vi "tester 2.vi"() -> ()   [LabVIEW 2020]
uses:
  VNA-Addresses.ctl
  <vilib>/Instr/_visa.llb/VISA Configure Serial Port (Instr).vi
panel:
  out "unsigned byte array 3":u8[](array[numeric])
  out "*(type *) &x 4":u64
  out "unsigned byte array 4":u8[](array[numeric]) format="%x"
  in  "byte order (0:big-endian, network order)":T1(ring)=enum."little-endian"
  out "*(type *) &x 3":u64
  out "*(type *) &x 2":u64
  in  "s":bool
  in  "unsigned byte array 2":u8[](array[numeric]) format="%x"
  out "unsigned byte array":u8[](array[numeric]) format="%x"
  out "Respons hex 2":u64 format="%x"
  out "length":i32
  out "XY Graph":cluster{i32[], dbl[]}[](graph)
  in  "y":bool
  out "Array":T2(array[cluster])
  in  "Command 2":i32 format="%x"
  in  "Write free":bool
  out "CMDADDR":u64 format="%x"
  out "*(type *) &x":u64
  out "data to write":u64 format="%x"
  in  "Read/write":bool
  in  "Address":T3
  in  "DAta to Write":u64
  out "bytes at port last":u32
  out "error out":errorcluster
  out "read buffer":string
  out "command worked":bool
  in  "clear command flag":bool
  out "Response string":string
  out "Respons hex":u64 format="%x"
  in  "Stop":bool
  in  "Write cmd":bool
  out "bytes at port":u32
  out "reading":bool
  out "Command":string="*IDN?"
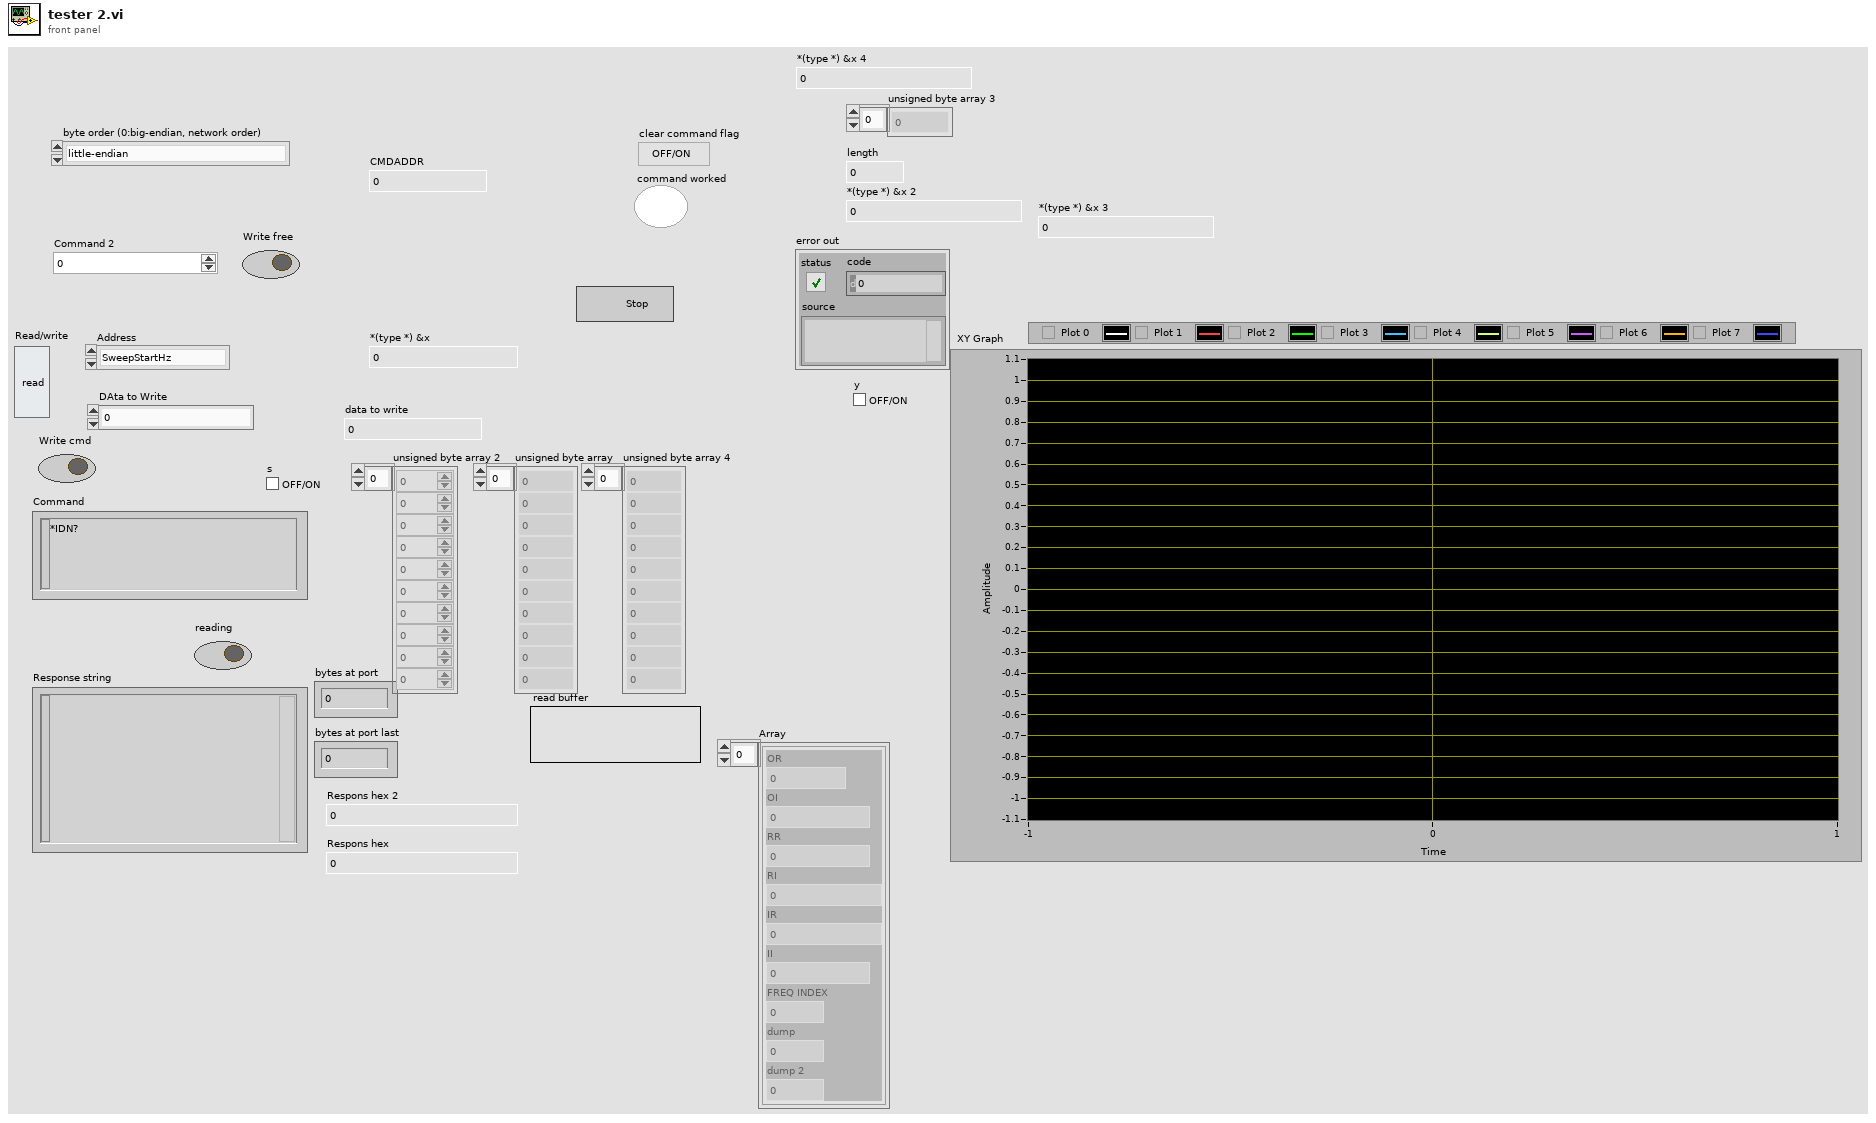
[diagram p1: front panel]
types:
  T1 = enum16{"big-endian, network order", "native, host order", "little-endian"}
  T2 = cluster{"OR":i32, "OI":i32, "RR":i32, "RI":i32, "IR":i32, "II":i32, "FREQ INDEX":u16, "dump":u16, "dump 2":u32}[]
  T3 = typedef "VNA-Addresses.ctl" = enum16{"SweepStartHz", "SweepStopHz", "SweepPoints", "valuesPerFrequency", "RawSamplesMode", "ValuesFIFO", "deviceVariant", "protocolVersion", "hardwareRevision", "firmwareMajor", "firmwareMinor"}
  T4 = cluster{"baud rate":u32, "data bits":u16, "parity":enum16{"None", "Odd", "Even", "Mark", "Space"}, "stop bits":u16, "flow control":u16}
  T5 = typedef "VNA-Commands.ctl" = enum16{"Nop", "Indicate", "Read 1B", "Read 2B", "Read 4B", "Read 8B", "Read FIFO", "Write 1B", "Write 2B", "Write 4B", "Write 8B", "Write FIFO"}
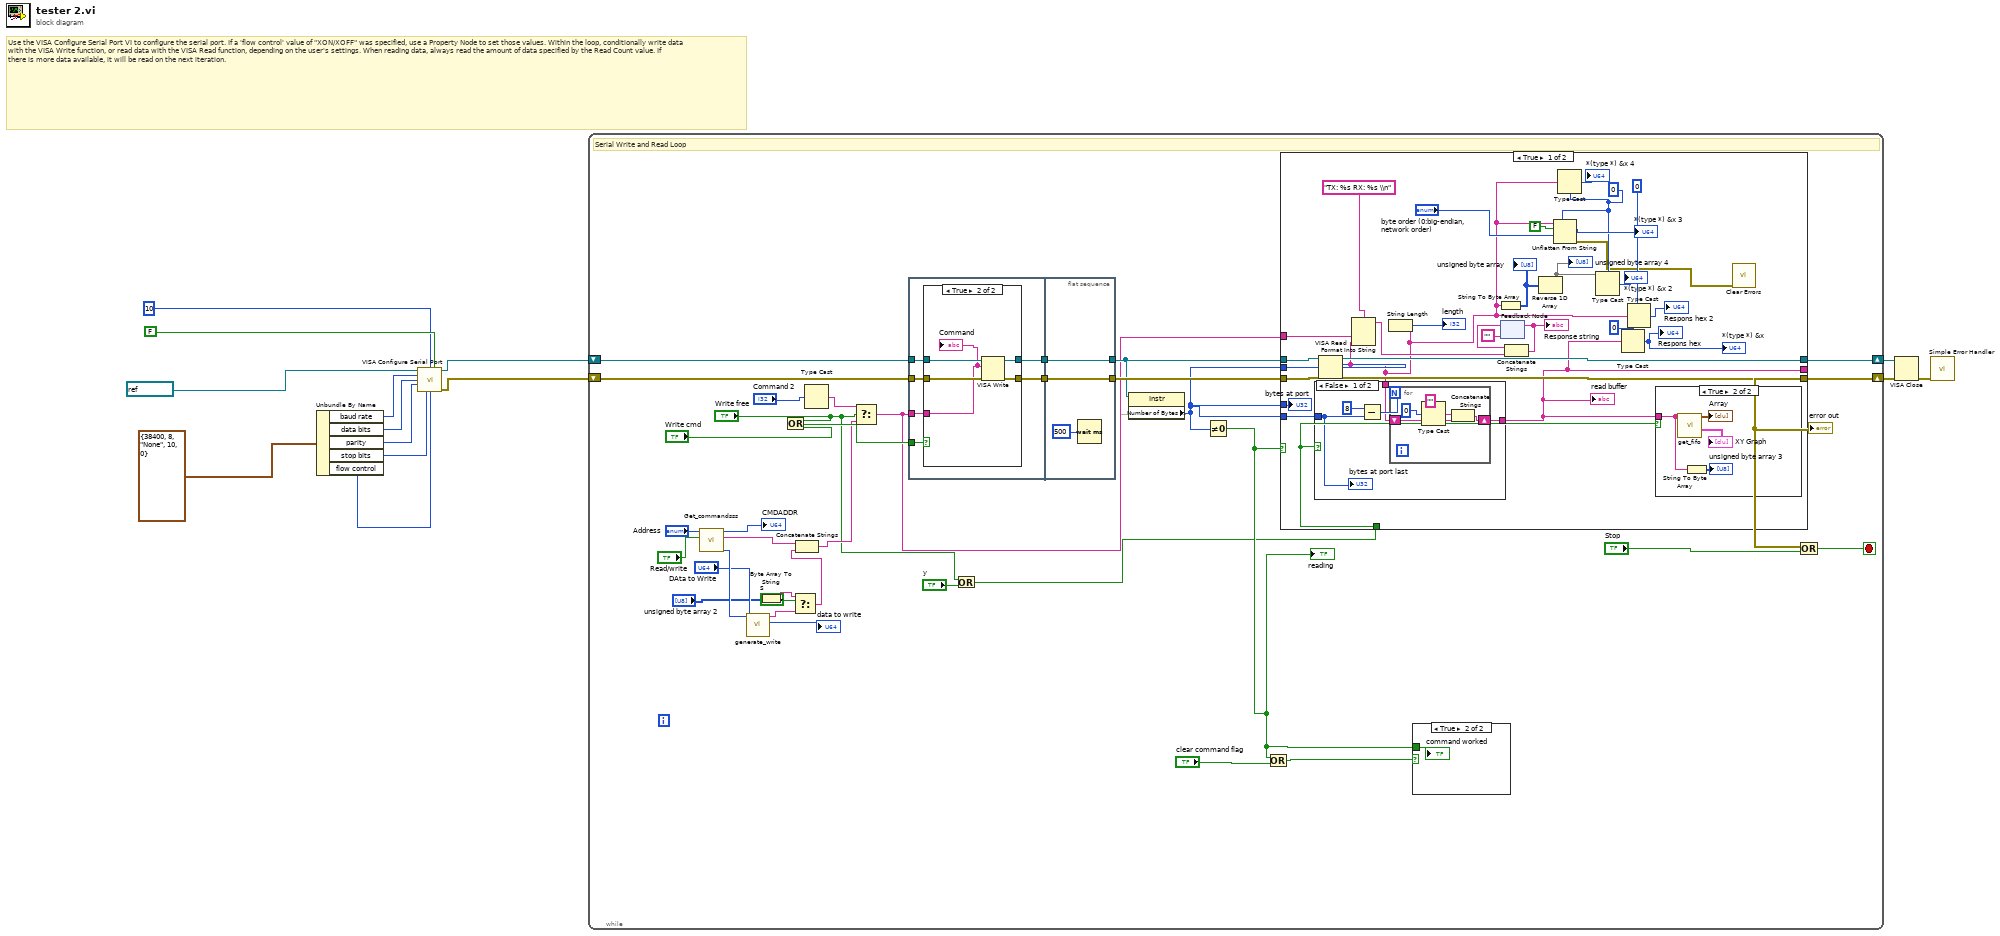
[diagram p0: block diagram]
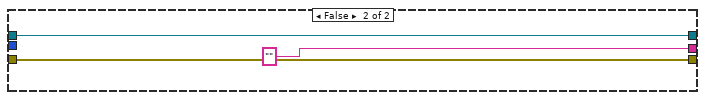
[diagram p6: hidden frame]
diagram:
  # "Use the VISA Configure Serial Port VI to configure the serial port. If a 'flow control' value of \"XON/XOFF\" was specified, use a Property Node to set those values. Within the loop, conditionally write data with the VISA Write function, or read data with the VISA Read function, depending on the user's settings. When reading data, always read the amount of data specified by the Read Count value. If there is more data available, it will be read on the next iteration."
  n1 = Unbundle By Name(T4 {"baud rate"=38400, "data bits"=8, "parity"=enum."None", "stop bits"=10, "flow control"=0} ("Serial Settings")) -> ("baud rate"=w7:u32, "data bits"=w8:u16, "parity"=w9:enum16{"None", "Odd", "Even", "Mark", "Space"}, "stop bits"=w10:u16, "flow control"=w4:u16)
  n2 = call-poly "VISA Configure Serial Port"("VISA resource name"=refnum<visa-resource-name> "COM5", "termination char\n(0xA = '\\n' = LF)"=u8 10 ("Termination Character"), "Enable Termination\nChar (T)"=FALSE ("End Read on Termination Character?"), "baud rate (9600)"=w7, "data bits (8)"=w8, "parity (0:none)"=w9, "stop bits (10: 1 bit)"=w10, "flow control (0:none)"=w4) -> ("VISA resource name out"=w2:refnum<visa-resource-name>, "error out"=w1:errorcluster)  [unwired: 2 in, 4 out]
  n3 = while {
    shift-right: [w49] -> w12
    shift-left: w2 -> [w48]
    shift-right: [w44] -> w13
    shift-left: w1 -> [w47]
    stop <- w45 stop-if-true
    # "Serial Write and Read Loop"
    n4 = call "Get_commandsss.vi"("Vertical Slide Switch"="Read/write", "Address"="Address") -> ("Command"=w35:T5, "CMDADDR string"=w36:string, "CMDADDR"=→"CMDADDR":u64)  [unwired: 7 in]
    n5 = call "generate_write.vi"("to Write"="DAta to Write", "Command"=w35) -> ("data to write"=→"data to write":u64, "data to write string"=w19:string)  [unwired: 8 in]
    n6 = Byte Array To String(unsigned byte array="unsigned byte array 2") -> (string=w18:string)
    n7 = Or(x="Write free", y="Write cmd") -> (x .or. y?=w28:bool)
    n8 = Select(t=w18, s="s", f=w19) -> (s? t:f=w16:string)
    n9 = Concatenate Strings(w36, w16) -> (w27:string)
    n10 = Type Cast(x="Command 2") -> (*(type *) &x=w26:string)  [unwired: 1 in]
    n11 = Select(t=w26, s="Write free", f=w27) -> (s? t:f=w24:string)
    n12 = flat-sequence {
      tunnel: w48 -> [w56]
      tunnel: w47 -> [w55]
      tunnel: w28 -> [w52]
      tunnel: w24 -> [w51]
      tunnel: [w54] -> w42
      tunnel: [w53] -> w41
      tunnel: [w65] -> w46
      tunnel: [w66] -> w40
      tunnel: w42 -> [w66]
      tunnel: w41 -> [w65]
      frame #0 {
        n13 = case shown="True" w52 {
          tunnel: w56 -> [w58 w63]
          tunnel: w55 -> [w57 w62]
          tunnel: [w58 w61] -> w54
          tunnel: [w57 w60] -> w53
          tunnel: w51 -> [_ w59]
          frame False {
          }
          frame True {
            n14 = VISA Write(VISA resource name=w63, write buffer=w59, error in (no error)=w62) -> (VISA resource name out=w61:refnum<visa-resource-name>, error out=w60:errorcluster)  [unwired: 1 out]
            "Command" <- w59
          }
        }
      }
      frame #1 {
        n15 = Wait (ms)(milliseconds to wait=u32 500) -> ()  [unwired: 1 out]
      }
    }
    n16 = Or(x="Write free", y="y") -> (x .or. y?=w22:bool)
    n17 = property class="Instr"(reference=w40) -> ("Serial Settings:Number of Bytes at Serial Port"=w15:u32)  [unwired: 1 in, 2 out]
    n18 = Not Equal To 0?(x=w15) -> (x != 0?=w37:bool)
    "reading" <- w37
    n19 = Or(x=w37, y="clear command flag") -> (x .or. y?=w39:bool)
    n20 = case shown="True" w37 {
      tunnel: [w94 w114] -> w49
      tunnel: w40 -> [w96 w114]
      tunnel: [w93 w113] -> w44
      tunnel: w46 -> [w95 w113]
      tunnel: w15 -> [w89 _]
      tunnel: [w82 "" ("read buffer")] -> _
      tunnel: w24 -> [w84 _]
      tunnel: w15 -> [w83 _]
      tunnel: w22 -> [w81 _]
      tunnel: w15 -> [w68 _]
      frame True {
        w70 = u64 0 ("Numeric")
        n21 = VISA Read(VISA resource name=w96, byte count=w89, error in (no error)=w95) -> (VISA resource name out=w94:refnum<visa-resource-name>, read buffer=w69:string, error out=w93:errorcluster)  [unwired: 1 out]
        n22 = case shown="False" w81 {
          tunnel: w83 -> [w101 _]
          tunnel: w69 -> [w98 w107]
          tunnel: [w97 w107] -> w82
          frame False {
            n23 = Subtract(x=u32 8, y=w101) -> (x-y=w99:u32)
            n24 = for {
              N: w99 -> [_]
              shift-right: [w105] -> w97
              shift-left: w98 -> [w106]
              n25 = Type Cast(type="", x=u8 0) -> (*(type *) &x=w102:string)
              n26 = Concatenate Strings(w102, w106) -> (w105:string)
            }
            "bytes at port last" <- w101
          }
          frame True {
          }
        }
        "read buffer" <- w82
        n27 = Format Into String(format string="TX: %s RX: %s \\n", w84, w69) -> (resulting string=w85:string)  [unwired: 2 in, 1 out]
        n28 = String Length(string=w69) -> (length=→"length":i32)
        n29 = String To Byte Array(string=w69) -> (unsigned byte array=w74:u8[])
        "unsigned byte array" <- w74
        n30 = feedback #1("") -> (w92:string)
        n31 = Concatenate Strings(w92, w85) -> (w91:string)
        "Response string" <- w91
        n32 = feedback-in #1(w91) -> ()
        n33 = Reverse 1D Array(array=w74) -> (reversed array=w73:u8[])
        "unsigned byte array 4" <- w73
        n34 = Unflatten From String(type=w70, binary string=w69, data includes array or string size? (T)=FALSE, byte order (0:big-endian, network order)="byte order (0:big-endian, network order)") -> (value=→"*(type *) &x 3":u64, error out=w67:errorcluster)  [unwired: 1 in, 1 out]
        n35 = Type Cast(type=w70, x=w69) -> (*(type *) &x=→"*(type *) &x 4":u64)
        n36 = Type Cast(type=w70, x=w73) -> (*(type *) &x=→"*(type *) &x 2":u64)
        n37 = Type Cast(type=u64 0 ("Numeric"), x=w82) -> (*(type *) &x=→"Respons hex" →"*(type *) &x":u64)
        n38 = Type Cast(type=u64 0 ("Numeric"), x=w69) -> (*(type *) &x=→"Respons hex 2":u64)
        n39 = case shown="True" w81 {
          tunnel: w82 -> [_ w109]
          frame False {
          }
          frame True {
            n40 = call "get_fifo.vi"("FIFO"=w109) -> ("XY Graph"=→"XY Graph":cluster{i32[], dbl[]}[], "Array"=→"Array":T2)  [unwired: 9 in]
            n41 = String To Byte Array(string=w109) -> (unsigned byte array=→"unsigned byte array 3":u8[])
          }
        }
        n42 = call <vilib>:"Clear Errors.vi"("error in (no error)"=w67) -> ()  [unwired: 5 in, 2 out]
        "bytes at port" <- w68
      }
      frame False {
      }
    }
    "error out" <- w44
    n43 = case shown="True" w39 {
      tunnel: w37 -> [_ w50]
      frame False {
      }
      frame True {
        "command worked" <- w50
      }
    }
    n44 = Or(x=w44, y="Stop") -> (x .or. y?=w45:bool)
  }
  n45 = VISA Close(VISA resource name=w12, error in (no error)=w13) -> (error out=w14:errorcluster)
  n46 = call <vilib>:"Simple Error Handler.vi"("error in (no error)"=w14) -> ()  [unwired: 1 in, 8 out]
